vi "Get_AVPP_instance.vi"(8 "error in (no error)":errorcluster, 11 "Gserver in":refnum<class "Gserver.lvclass">) -> (0 "error out":errorcluster, 2 "AVPP class":refnum<data-value>, 3 "Gserver out":refnum<class "Gserver.lvclass">)   [LabVIEW 2014, in "Gserver.lvclass"]
doc: "Get AVPP object reference.\nThis method is intended to allow HISW to get access to the AVPP instance.\nThis AVPP instance holds the FAMM instance and can therefore access the historian memory."
uses:
  Gserver.lvclass
  AVPP/AVPP.lvclass
  Gserver.lvclass/Gserver.ctl
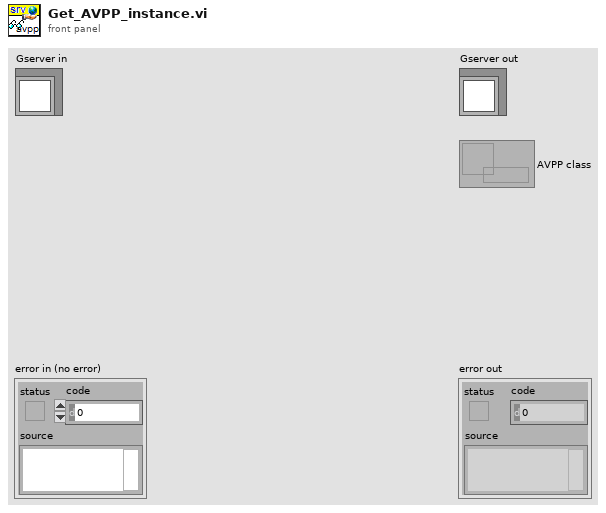
[diagram p1: front panel]
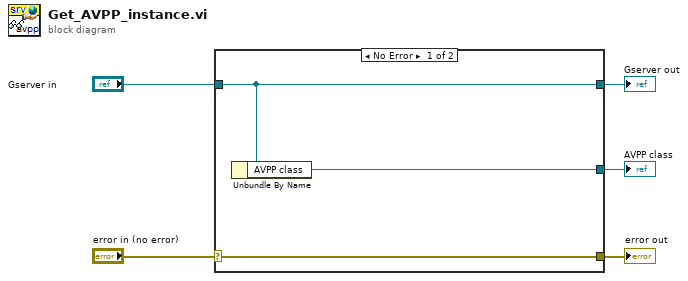
[diagram p0: block diagram]
diagram:
  n1 = case shown="No Error" "error in (no error)" {
    selector: "error in (no error)" -> [w8 w9]
    tunnel: [w8 w9] -> w4
    tunnel: [w7 w10] -> w2
    tunnel: "Gserver in" -> [w7 w10]
    tunnel: [w6 _] -> w1
    frame No Error {
      n2 = Unbundle By Name(w7) -> ("AVPP class"=w6:refnum<data-value>)
    }
    frame Error {
    }
  }
  "error out" <- w4
  "Gserver out" <- w2
  "AVPP class" <- w1
